vi "Line Align&Snap 90.vi"(9 "LA limit throt wheel":dbl=0.6, 10 "LA limit throttle":dbl=1.0) -> (1 "Right":dbl, 2 "Left":dbl)   [LabVIEW 2018]
uses:
  <vilib>/addons/control/pid/pid.llb/PID (DBL).vi
  <vilib>/addons/control/pid/NI_PID_pid.lvlib
panel:
  in  "offset":dbl
  out "Snap 90":cluster{"Snap Goal":dbl, "setpoint":dbl}(graph)
  in  "Turn Low PID gains 4":T1={"proportional gain (Kc)"=0.018, "integral time (Ti, min)"=1.0, "derivative time (Td, min)"=0.0018000000000000004} {"derivative time (Td, min)" format="%.4f"; "integral time (Ti, min)" format="%.4f"; "proportional gain (Kc)" format="%.4f"}
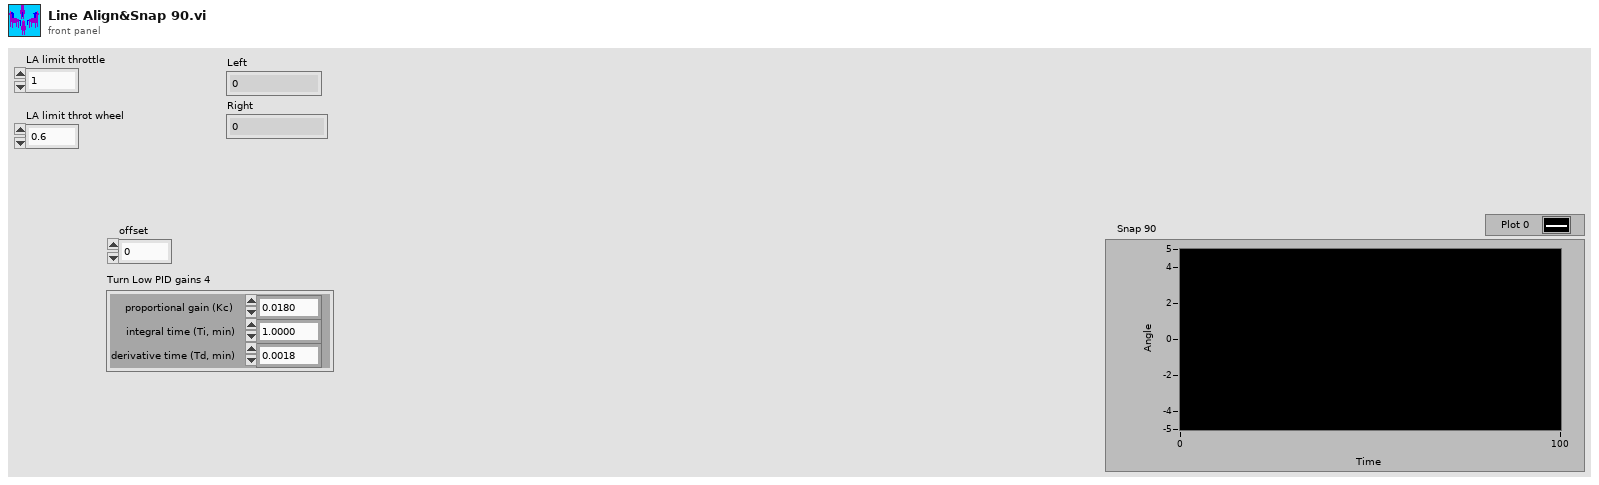
[diagram p1: front panel]
types:
  T1 = cluster{"proportional gain (Kc)":dbl, "integral time (Ti, min)":dbl, "derivative time (Td, min)":dbl}
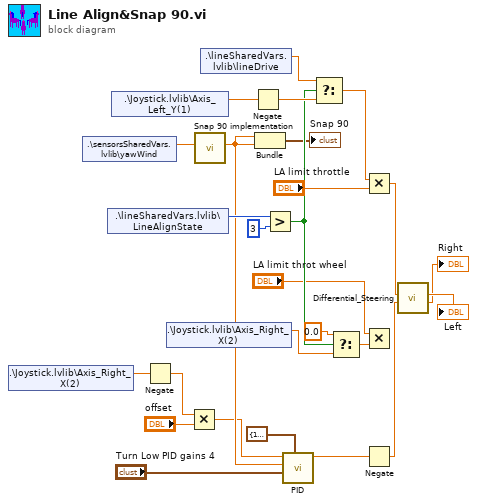
[diagram p0: block diagram]
diagram:
  n1 = shared-variable ".\\Joystick.lvlib\\Axis_Right_X(2)"() -> (w6:dbl)  [unwired: 1 in, 1 out]
  n2 = shared-variable ".\\sensorsSharedVars.lvlib\\yawWind"() -> (w3:dbl)  [unwired: 1 in, 1 out]
  n3 = shared-variable ".\\lineSharedVars.lvlib\\LineAlignState"() -> (w26:i32)  [unwired: 1 in, 1 out]
  n4 = shared-variable ".\\Joystick.lvlib\\Axis_Left_Y(1)"() -> (w23:dbl)  [unwired: 1 in, 1 out]
  n5 = Negate(x=w6) -> (-x=w4:dbl)
  n6 = shared-variable ".\\Joystick.lvlib\\Axis_Right_X(2)"() -> (w16:dbl)  [unwired: 1 in, 1 out]
  n7 = Multiply(x=w4, y="offset") -> (x*y=w5:dbl)
  n8 = call "Snap 90 implementation.vi"("YawWrap"=w3) -> ("Snap Goal"=w7:dbl)  [unwired: 10 in]
  n9 = shared-variable ".\\lineSharedVars.lvlib\\lineDrive"() -> (w24:dbl)  [unwired: 1 in, 1 out]
  n10 = Negate(x=w23) -> (-x=w21:dbl)
  n11 = Bundle("Snap Goal"=w7, "Snap Goal"=w7) -> (→"Snap 90":cluster{"Snap Goal":dbl, "Snap Goal":dbl})  [unwired: 1 in]
  n12 = Greater?(x=w26, y=3) -> (0:w19:bool)
  n13 = call-poly <vilib>:"PID.vi"("output range"=cluster{"output high":dbl, "output low":dbl} {"output high"=1.0, "output low"=-1.0}, "PID gains"="Turn Low PID gains 4", "process variable"=w7, "setpoint"=w5) -> ("output"=w14:dbl)  [unwired: 6 in, 1 out]
  n14 = Select(t=w24, s=w19, f=w21) -> (s? t:f=w20:dbl)
  n15 = Select(t=0.0, s=w19, f=w16) -> (s? t:f=w18:dbl)
  n16 = Multiply(x=w20, y="LA limit throttle") -> (x*y=w11:dbl)
  n17 = Multiply(x="LA limit throt wheel", y=w18) -> ()  [unwired: 1 out]
  n18 = Negate(x=w14) -> (-x=w10:dbl)
  n19 = call <userlib>:"Differential_Steering.vi"("Steer"=w10, "Base"=w11) -> ("Right"=→"Right":dbl, "Left"=→"Left":dbl)  [unwired: 4 in]
